vi "Ping Result.vi"(8 "error in (no error)":errorcluster, 11 "Network Test in":refnum<class "Network Test.lvclass">) -> (0 "error out":errorcluster, 3 "Network Test out":refnum<class "Network Test.lvclass">)   [LabVIEW 2017, in "Network Test.lvlib" / "Network Test.lvclass"]
uses:
  Network Test.lvclass
  Ping Test Configuration.ctl
  Network Test.lvlib
panel:
  in  "Ping Test":T1
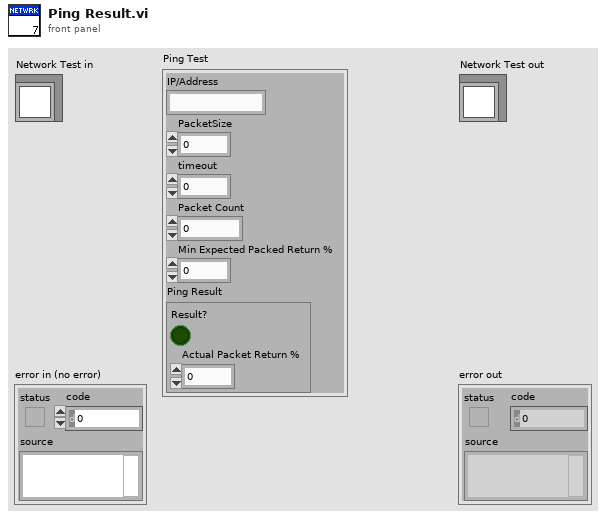
[diagram p1: front panel]
types:
  T1 = typedef "Network Test.lvlib/Ping Test Configuration.ctl" = cluster{"IP/Address":string, "PacketSize":i32, "timeout":i32, "Packet Count":i32, "Min Expected Packed Return %":dbl, "Ping Result":cluster{"Result?":bool, "Actual Packet Return %":dbl}}
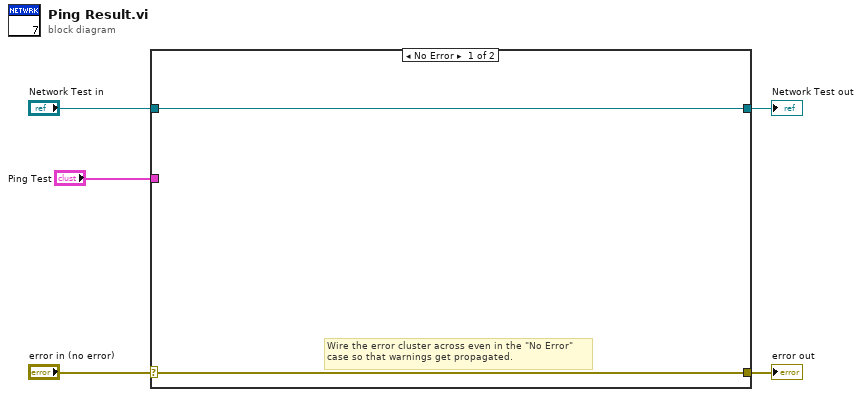
[diagram p0: block diagram]
diagram:
  n1 = case shown="No Error" "error in (no error)" {
    selector: "error in (no error)" -> [w6 w9]
    tunnel: [w6 w9] -> w4
    tunnel: [w7 w8] -> w2
    tunnel: "Network Test in" -> [w7 w8]
    tunnel: "Ping Test" -> [_ _]
    frame No Error {
      # "Wire the error cluster across even in the \"No Error\"\ncase so that warnings get propagated."
    }
    frame Error {
    }
  }
  "error out" <- w4
  "Network Test out" <- w2
